vi "Data_Acquisition log.vi"() -> ()   [LabVIEW 2020]
uses:
  Classes/Smart Eye Pro Drivers/Data Class/Datatypes/Data_AllInOne_class/Attribute.vi
  Classes/Smart Eye Pro Drivers/Decode Class/Decode_Packet/Decode_type.ctl
  Global Variables/Time_Trigger.vi
  Global Variables/Global Enable Logging.vi
  Classes/Smart Eye Pro Drivers/SmartEyeProDriver_class/SmartEyeProDriver.lvclass
  Classes/Smart Eye Pro Drivers/Data Class/Datatypes/Data_AllInOne_class/Data_AllInOne.lvclass
  Classes/Smart Eye Pro Drivers/Decode Class/Decode_Packet/Decode_Packet.lvclass
panel:
  out "Enable Logging":bool
  out "appended array 2":dbl[](array[numeric])
  out "appended array":dbl[](array[numeric])
  out "size(s)":i32[](array[numeric])
  out "History":dbl[][](array[numeric])
  out "error out 2":errorcluster
  out "Attribute 2":T1
  in  "stop 2":bool
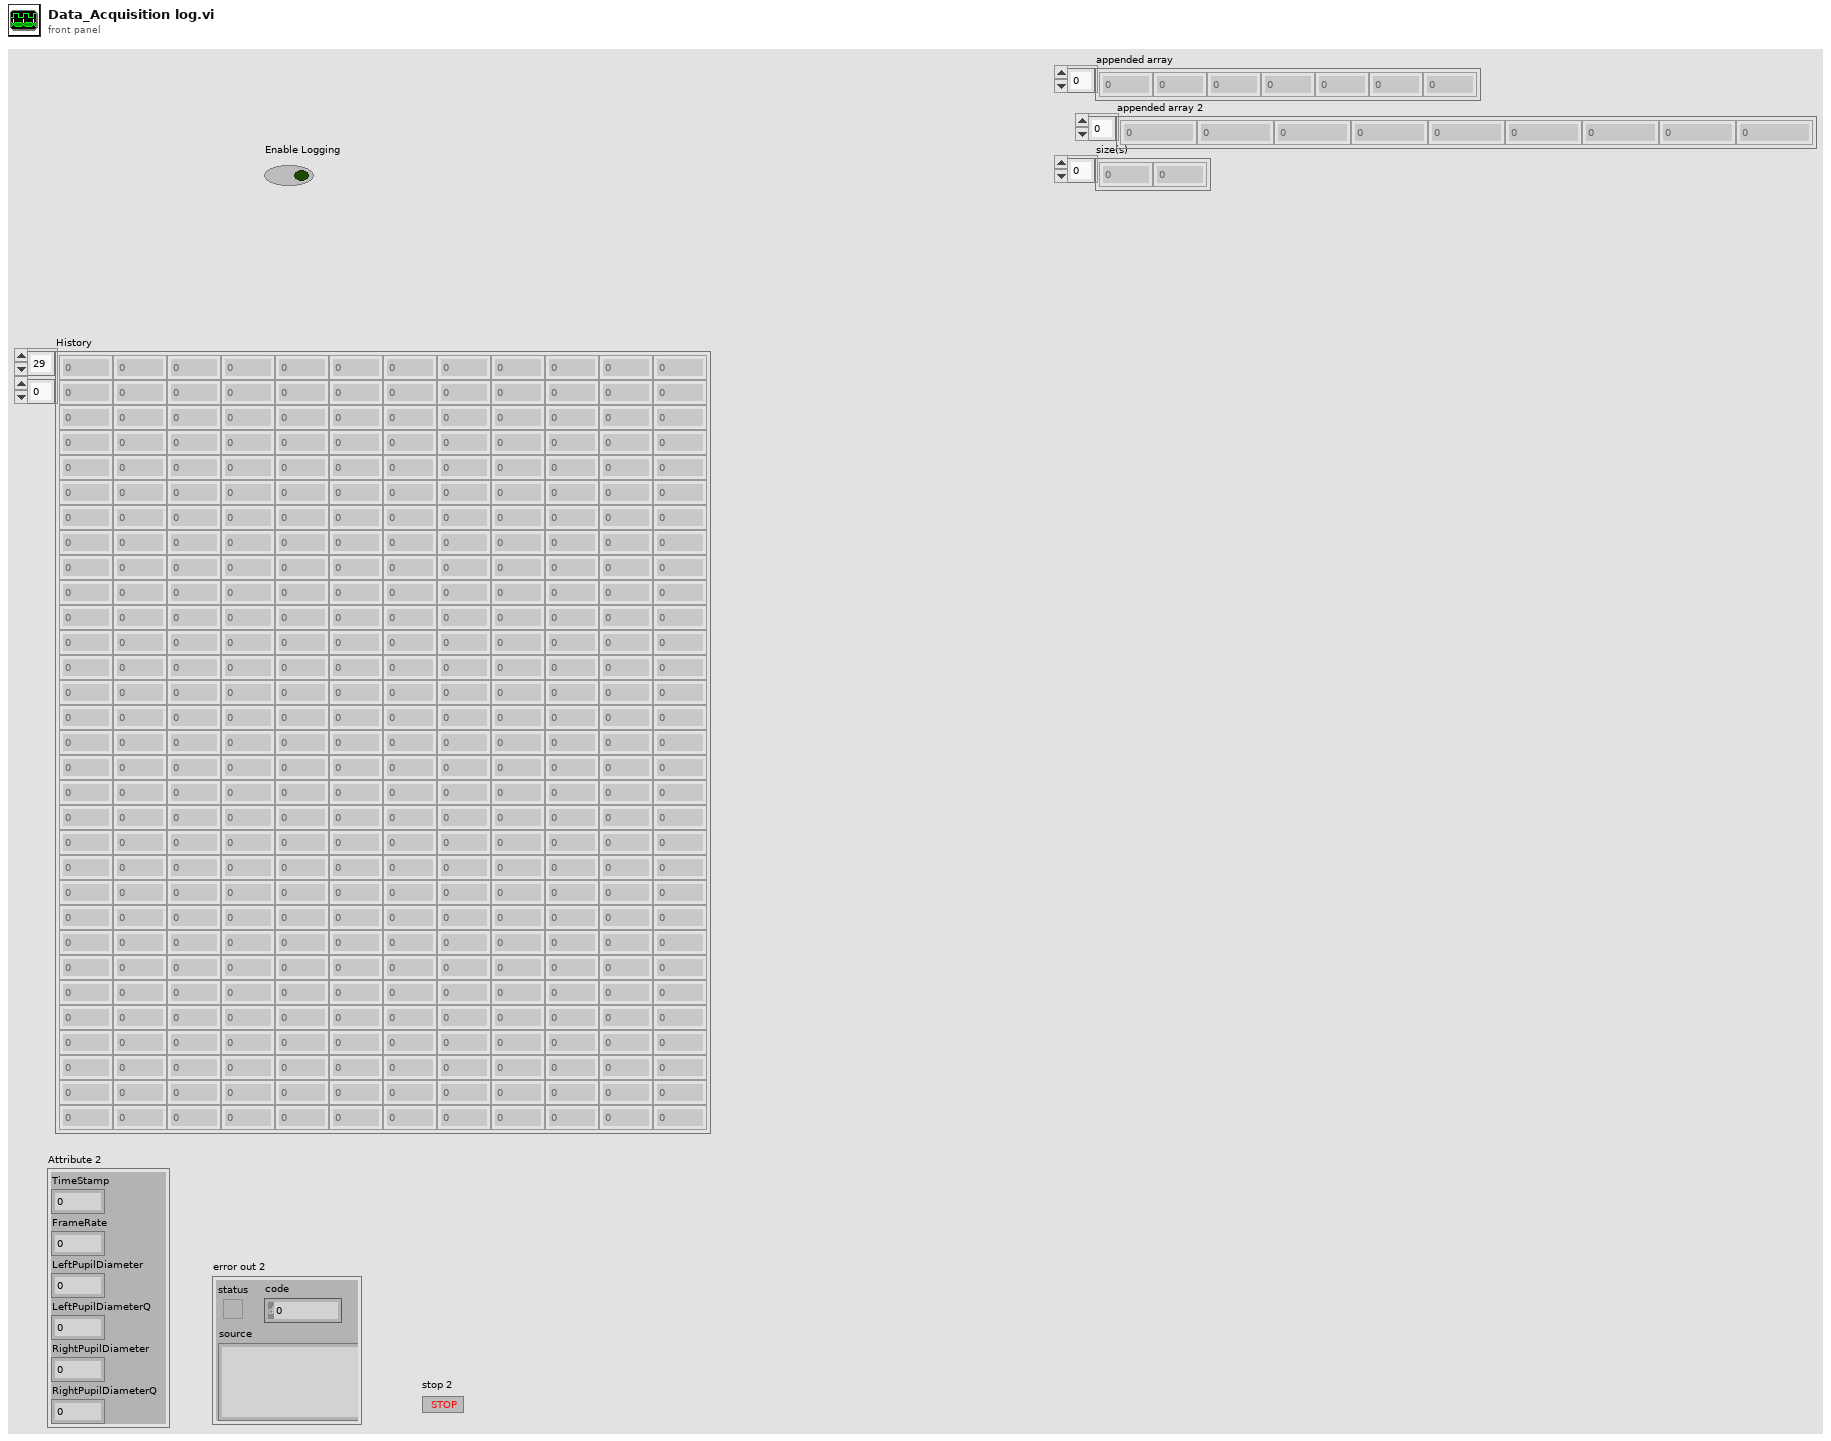
[diagram p1: front panel]
types:
  T1 = typedef "Data_AllInOne.lvclass/Attribute.vi" = cluster{"TimeStamp":u64, "FrameRate":dbl, "LeftPupilDiameter":dbl, "LeftPupilDiameterQ":dbl, "RightPupilDiameter":dbl, "RightPupilDiameterQ":dbl}
  T2 = enum16{"big-endian, network order", "native, host order", "little-endian"}
  T3 = typedef "Decode_Packet.lvclass/Decode_type.ctl" = enum16{"Frame Information", "Raw Gaze", "Pupilometry", "All In One"}
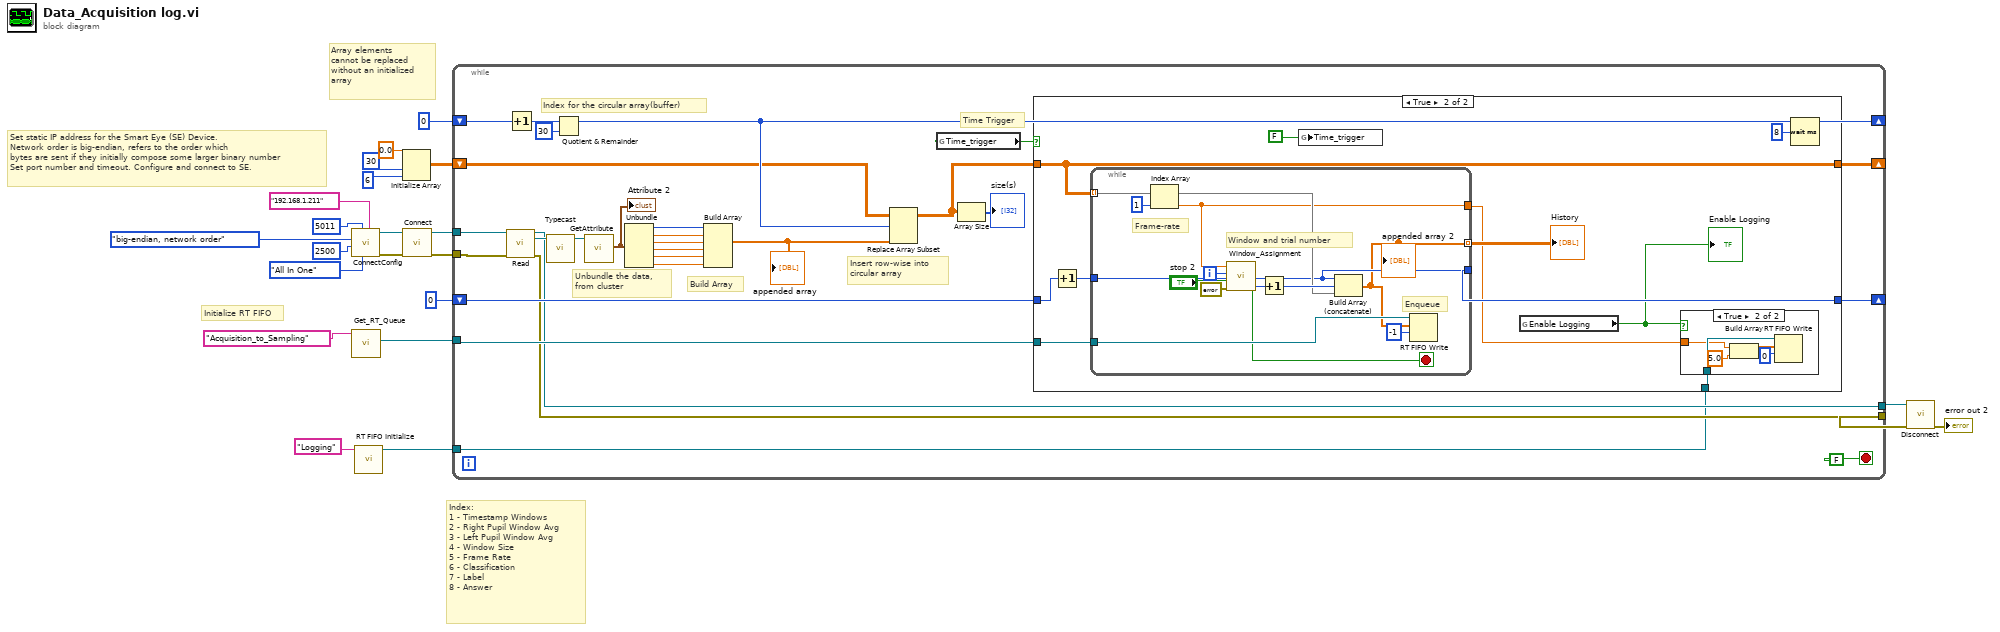
[diagram p0: block diagram]
diagram:
  # "Array elements \ncannot be replaced \nwithout an initialized \narray"
  # "Index: \n1 - Timestamp Windows \n2 - Right Pupil Window Avg \n3 - Left Pupil Window Avg\n4 - Window Size\n5 - Frame Rate\n6 - Classification\n7 - Label \n8 - Answer"
  # "Initialize RT FIFO"
  # "Set static IP address for the Smart Eye (SE) Device. \nNetwork order is big-endian, refers to the order which \nbytes are sent if they initially compose some larger binary number\nSet port number and timeout. Configure and connect to SE."
  n1 = call "ConnectConfig.vi"("service name"="192.168.1.211", "Decode type"=Decode_type."All In One", "port"=u16 5011, "timeout ms (25000)"=2500, "byte order (0:big-endian, network order)"=T2."big-endian, network order") -> ("error out"=w21:errorcluster, "Smart_Eye_Pro_Driver out"=w22:refnum<class "SmartEyeProDriver.lvclass">)  [unwired: 5 in]
  n2 = call "Get_RT_Queue.vi"("String"="Acquisition_to_Sampling") -> ("rt fifo double"=w11:refnum<k33>)  [unwired: 8 in, 2 out]
  n3 = call "RT FIFO Initialize.vi"("name (unnamed)"="Logging") -> ("rt fifo"=w5:refnum<k33>)  [unwired: 9 in, 1 out]
  n4 = Initialize Array(0.0 ("element"), 30 ("dimension size"), 6 ("dimension size")) -> (w1:dbl[][])
  n5 = call "Connect.vi"("error in (no error)"=w21, "Smart_Eye_Pro_Driver in"=w22) -> ("error out"=w14:errorcluster, "Smart_Eye_Pro_Driver out"=w15:refnum<class "SmartEyeProDriver.lvclass">)  [unwired: 8 in]
  n6 = while {
    tunnel: w15 -> [w41]
    tunnel: w14 -> [w40]
    shift-right: [w36] -> _
    shift-left: 0 -> [w39]
    shift-right: [w28] -> _
    shift-left: w1 -> [w35]
    tunnel: w11 -> [w33]
    shift-right: [w31] -> _
    shift-left: 0 -> [w32]
    tunnel: [w30] -> w8
    tunnel: [w29] -> w7
    tunnel: w5 -> [w23]
    stop <- FALSE stop-if-true
    # "Time Trigger"
    # "Insert row-wise into \ncircular array"
    # "Build Array"
    # "Unbundle the data, \nfrom cluster"
    # "Index for the circular array(buffer)"
    n7 = call "Read.vi"("Smart_Eye_Pro_Driver in"=w41, "error in (no error)"=w40) -> ("Smart_Eye_Pro_Driver out"=w30:refnum<class "SmartEyeProDriver.lvclass">, "Data out"=w50:refnum<class "Data.lvclass">, "error out"=w29:errorcluster)  [unwired: 8 in, 3 out]
    n8 = Increment(x=w39) -> (x+1=w38:i32)
    n9 = call "Typecast.vi"("Data in"=w50) -> ("Data_Gaze out"=w49:refnum<class "Data_AllInOne.lvclass">)  [unwired: 9 in, 1 out]
    n10 = Quotient & Remainder(x=w38, y=30 ("floor(x/y)")) -> (x-y*floor(x/y)=w36:i32)  [unwired: 1 out]
    n11 = call "GetAttribute.vi"("Data_AllInOne in"=w49) -> ("Attribute"=w43:T1)  [unwired: 8 in, 2 out]
    "Attribute 2" <- w43
    n12 = Unbundle(w43) -> ("TimeStamp"=w44:u64, "FrameRate"=w42:dbl, "LeftPupilDiameter"=w45:dbl, "LeftPupilDiameterQ"=w46:dbl, "RightPupilDiameter"=w47:dbl, "RightPupilDiameterQ"=w48:dbl)
    n13 = Build Array(w44, w42, w45, w46, w47, w48) -> (w34:dbl[])
    "appended array" <- w34
    n14 = Replace Array Subset(array=w35, new element=w34, index (row)=w36) -> (w24:dbl[][])  [unwired: 1 in]
    n15 = global read "Time_Trigger.vi" "Time_trigger"() -> (w26:bool)
    n16 = Array Size(array=w24) -> (size(s)=→"size(s)":i32[])
    n17 = case shown="True" w26 {
      tunnel: w24 -> [w52 w60]
      tunnel: [w52 w60] -> w28
      tunnel: w33 -> [_ w63]
      tunnel: w32 -> [w51 w62]
      tunnel: [w51 w59] -> w31
      tunnel: w23 -> [_ w56]
      frame False {
      }
      frame True {
        n18 = Increment(x=w62) -> (x+1=w61:i32)
        n19 = while {
          tunnel: w63 -> [w81]
          tunnel: w60 -> [w74] mode=indexing
          tunnel: w61 -> [w72]
          tunnel: [w72] -> w59
          tunnel: [w71] -> w58 mode=indexing
          tunnel: [w70] -> w55
          i -> [w80]
          stop <- w77 stop-if-true
          # "Frame-rate"
          # "Enqueue"
          # "Window and trial number"
          n20 = Index Array(array=w74, index=1) -> (element=w70:dbl)
          n21 = call "Window_Assignment.vi"("error in (no error)"=errorcluster {"status"=FALSE, "code"=0, "source"=""}, "stop"="stop 2", "Iteration"=w80, "FrameRate"=w70) -> ("Stop Sample"=w77:bool, "Window Number"=w76:i64)  [unwired: 6 in]
          n22 = Increment(x=w76) -> (x+1=w75:i64)
          n23 = Build Array (concatenate)(w72, w75, w74) -> (w71:dbl[])
          "appended array 2" <- w71
          n24 = RT FIFO Write(0:w81, 1:w71, 2:-1 ("timeout in ms (0)")) -> ()  [unwired: 2 in, 4 out]
        }
        "History" <- w58
        n25 = global write "Time_Trigger.vi" "Time_trigger"(FALSE ("OK Button")) -> ()
        n26 = global read "Global Enable Logging.vi" "Enable Logging"() -> (w54:bool)
        "Enable Logging" <- w54
        n27 = case shown="True" w54 {
          tunnel: w56 -> [_ w65]
          tunnel: w55 -> [_ w64]
          frame False {
          }
          frame True {
            n28 = Build Array(w64, 5.0 ("element")) -> (w68:dbl[])
            n29 = RT FIFO Write(0:w65, 1:w68, 2:0 ("timeout in ms (0)")) -> ()  [unwired: 2 in, 4 out]
          }
        }
        n30 = Wait (ms)(milliseconds to wait=u32 8) -> ()  [unwired: 1 out]
      }
    }
  }
  n31 = call "Disconnect.vi"("error in (no error)"=w7, "Smart_Eye_Pro_Driver in"=w8) -> ("error out"=→"error out 2":errorcluster)  [unwired: 8 in, 1 out]
